vi "driveLoadingStationToCargoShipSM.vi"(9 "Initialized":bool) -> (2 "Drive State":T1)   [LabVIEW 2018]
uses:
  driveStateEnum.ctl
  driveLoadingStationToCargoShipEnum.ctl
  MotionProfile/Constants.vi
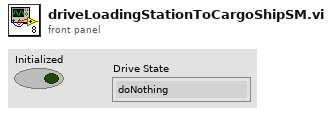
[diagram p1: front panel]
types:
  T1 = typedef "driveStateEnum.ctl" = enum16{"doNothing", "Manuel", "Teleop", "Follow Path (init)", "Follow Path", "Move to Target", "Climb", "Line Align", "Rotate180", "Align50Degrees"}
  T2 = typedef "driveLoadingStationToCargoShipEnum.ctl" = enum16{"1 - MP Back Up (init)", "2 - MP Back Up", "3 - Spin", "4 - MP Goto Cargo (init)", "5 - MP Goto Cargo", "6 - doNothing"}
  T3 = typedef "WPI_MotorControlDeviceRef.ctl" = cluster{"DeviceStatus":errorcluster, "Type":T4, "PWM":cluster{"PWM Channel":T5, "DeadBand":T6}, "CAN":cluster{"Device Number":u8, "SetOutput VI Ref":variant, "GetOutput VI Ref":variant, "Enable VI Ref":variant, "Disable VI Ref":variant, "Data":variant}, "Invert":bool, "DIO PWM":cluster{"PWM \"Enable\" Channel":T5, "DIOChannel":T7, "PWM Rate":dbl}}
  T4 = typedef "WPI_MotorControlType.ctl" = enum16{"PWM", "CAN", "DIO PWM"}
  T5 = typedef "FPGA_DIOPWMChannel.ctl" = enum8{"PWM 0", "PWM 1", "PWM 2", "PWM 3", "PWM 4", "PWM 5", "PWM 6", "PWM 7", "PWM 8", "PWM 9", "PWM MXP 0", "PWM MXP 1", "PWM MXP 2", "PWM MXP 3", "PWM MXP 4", "PWM MXP 5", "PWM MXP 6", "PWM MXP 7", "PWM MXP 8", "PWM MXP 9", "Invalid"}
  T6 = typedef "WPI_PWMDeadband.ctl" = cluster{"Name":string, "maxPositivePwm":i32, "minPositivePwm":i32, "centerPwm":i32, "maxNegativePwm":i32, "minNegativePwm":i32, "angularRange":u16}
  T7 = typedef "FPGA_DIOChannel.ctl" = enum8{"DIO 0", "DIO 1", "DIO 2", "DIO 3", "DIO 4", "DIO 5", "DIO 6", "DIO 7", "DIO 8", "DIO 9", "DIO MXP 0", "DIO MXP 1", "DIO MXP 2", "DIO MXP 3", "DIO MXP 4", "DIO MXP 5", "DIO MXP 6", "DIO MXP 7", "DIO MXP 8", "DIO MXP 9", "DIO MXP 10", "DIO MXP 11", "DIO MXP 12", "DIO MXP 13", "DIO MXP 14", "DIO MXP 15", "SPI Port CS1", "SPI Port CS2", "SPI Port CS3", "SPI Port MISO", "SPI Port MOSI", "Invalid"}
  T8 = enum16{"[0, 360]", "[-180, 180]", "[0, 2PI]", "[-PI, PI]"}
  T9 = typedef "CTRE_PigeonIMU_DeviceRef.ctl" = cluster{"DeviceStatus":errorcluster, "Device Number":u8, "Type":T10, "Device ID":u32, "Handle":u64, "UsageFrame":u32, "Library Path":path}
  T10 = typedef "CTRE_PigeonIMU_ConnectionType.ctl" = u32
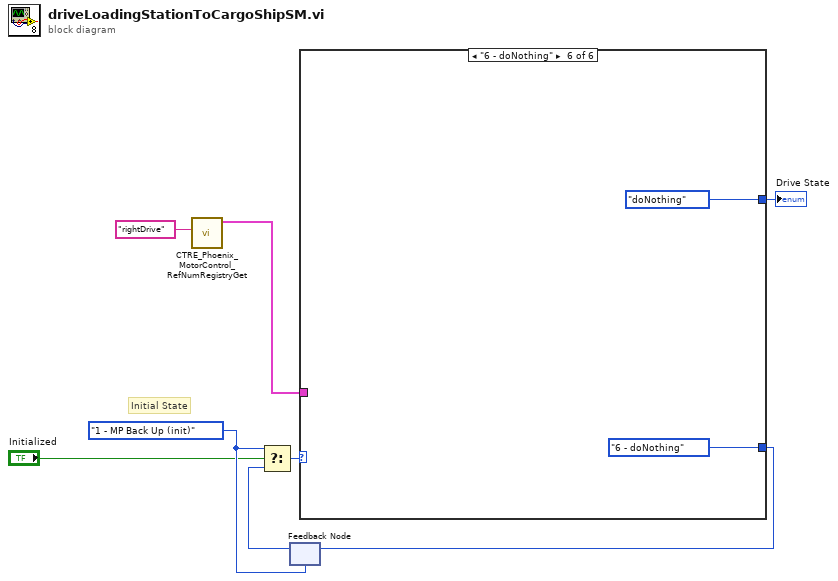
[diagram p0: block diagram]
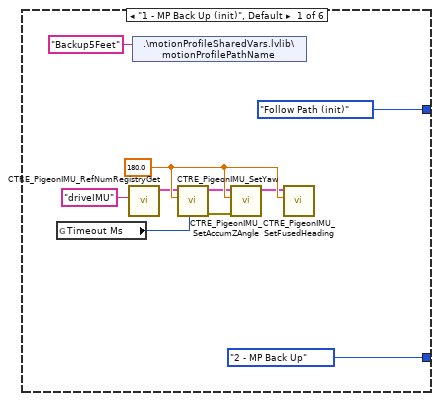
[diagram p2: hidden frame]
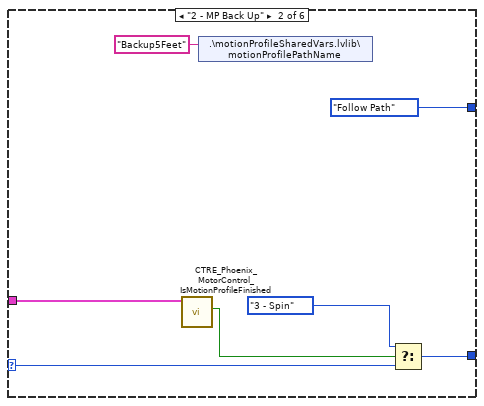
[diagram p3: hidden frame]
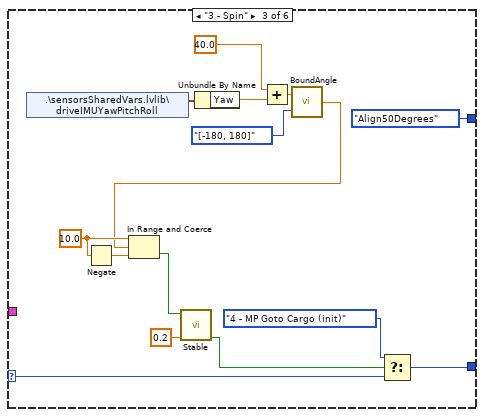
[diagram p4: hidden frame]
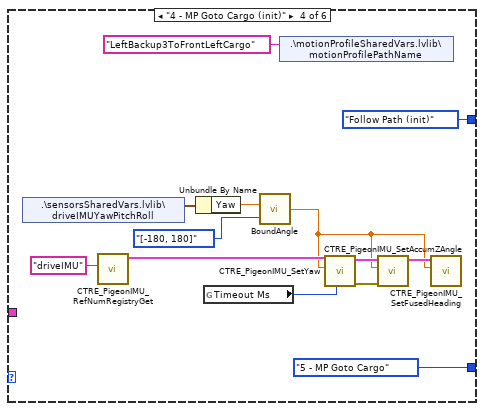
[diagram p5: hidden frame]
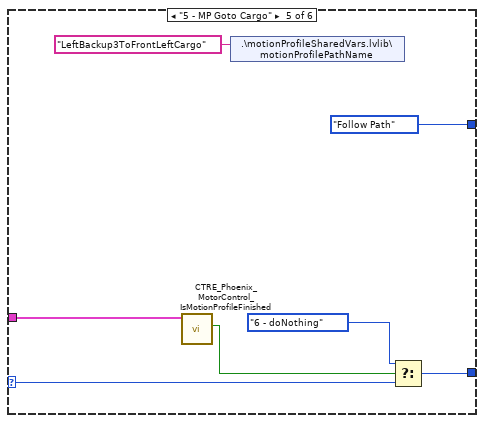
[diagram p6: hidden frame]
diagram:
  w6 = driveLoadingStationToCargoShipEnum."1 - MP Back Up (init)"
  # "Initial State"
  n1 = call <vilib>:"CTRE_Phoenix_MotorControl_RefNumRegistryGet.vi"("refnum name"="rightDrive") -> ("PhoenixMotorControlDevRef"=w3:T3)  [unwired: 9 in, 1 out]
  n2 = feedback #1(w6) -> (w7:T2)
  n3 = Select(t=w6, s="Initialized", f=w7) -> (s? t:f=w8:T2)
  n4 = case shown="\"6 - doNothing\"" w8 {
    selector: w8 -> [_ w20 w40 _ w55 _]
    tunnel: [driveLoadingStationToCargoShipEnum."2 - MP Back Up" w24 w39 driveLoadingStationToCargoShipEnum."5 - MP Goto Cargo" w59 driveLoadingStationToCargoShipEnum."6 - doNothing"] -> w5
    tunnel: [driveStateEnum."Follow Path (init)" ("Drive State Enum") driveStateEnum."Follow Path" ("Drive State Enum") driveStateEnum."Align50Degrees" ("Drive State Enum") driveStateEnum."Follow Path (init)" ("Drive State Enum") driveStateEnum."Follow Path" ("Drive State Enum") driveStateEnum."doNothing" ("Drive State Enum")] -> w1
    tunnel: w3 -> [_ w22 _ _ w57 _]
    frame "1 - MP Back Up (init)", Default {
      w15 = 180.0 ("Angle (Deg)")
      n5 = global read "Constants.vi" "Timeout Ms"() -> (w12:i32)
      n6 = call <vilib>:"CTRE_PigeonIMU_RefNumRegistryGet.vi"("refnum name"="driveIMU") -> ("PigeonIMUDevRef"=w9:T9)  [unwired: 9 in, 1 out]
      n7 = shared-variable ".\\motionProfileSharedVars.lvlib\\motionProfilePathName"("Backup5Feet" ("motionProfilePathName")) -> ()  [unwired: 1 in, 1 out]
      n8 = call <vilib>:"CTRE_PigeonIMU_SetYaw.vi"("timeoutMs"=w12, "Value"=w15, "PigeonIMUDevRef"=w9) -> ("error out"=w10:errorcluster, "PigeonIMUDevRef"=w11:T9)  [unwired: 7 in]
      n9 = call <vilib>:"CTRE_PigeonIMU_SetAccumZAngle.vi"("error in (no error)"=w10, "Angle (Deg)"=w15, "PigeonIMUDevRef"=w11) -> ("PigeonIMUDevRef"=w13:T9)  [unwired: 7 in, 1 out]
      n10 = call <vilib>:"CTRE_PigeonIMU_SetFusedHeading.vi"("Value"=w15, "PigeonIMUDevRef 2"=w13) -> ()  [unwired: 8 in, 2 out]
    }
    frame "2 - MP Back Up" {
      n11 = call <vilib>:"CTRE_Phoenix_MotorControl_IsMotionProfileFinished.vi"("PhoenixMotorControlDevRef"=w22) -> ("Is Motion Profile Finished?"=w21:bool)  [unwired: 8 in, 2 out]
      n12 = shared-variable ".\\motionProfileSharedVars.lvlib\\motionProfilePathName"("Backup5Feet" ("motionProfilePathName")) -> ()  [unwired: 1 in, 1 out]
      n13 = Select(t=driveLoadingStationToCargoShipEnum."3 - Spin", s=w21, f=w20) -> (s? t:f=w24:T2)
    }
    frame "3 - Spin" {
      w33 = 10.0 ("upper limit")
      n14 = shared-variable ".\\sensorsSharedVars.lvlib\\driveIMUYawPitchRoll"() -> (w32:cluster{"Yaw":dbl, "Pitch":dbl, "Roll":dbl})  [unwired: 1 in, 1 out]
      n15 = Negate(x=w33) -> (-x=w34:dbl)
      n16 = Unbundle By Name(w32) -> ("Yaw"=w27:dbl)
      n17 = Add(x=40.0 ("y"), y=w27) -> (x+y=w28:dbl)
      n18 = call <userlib>:"BoundAngle.vi"("Type"=T8."[-180, 180]", "Angle"=w28) -> ("Bound Angle"=w29:dbl)
      n19 = In Range and Coerce(upper limit=w33, x=w29, lower limit=w34) -> (In Range?=w35:bool)  [unwired: 1 out]
      n20 = call <userlib>:"Stable.vi"("Eval Period (sec)"=0.2, "Signal Input"=w35) -> ("Stable"=w37:bool)  [unwired: 9 in]
      n21 = Select(t=driveLoadingStationToCargoShipEnum."4 - MP Goto Cargo (init)", s=w37, f=w40) -> (s? t:f=w39:T2)
    }
    frame "4 - MP Goto Cargo (init)" {
      n22 = shared-variable ".\\sensorsSharedVars.lvlib\\driveIMUYawPitchRoll"() -> (w44:cluster{"Yaw":dbl, "Pitch":dbl, "Roll":dbl})  [unwired: 1 in, 1 out]
      n23 = call <vilib>:"CTRE_PigeonIMU_RefNumRegistryGet.vi"("refnum name"="driveIMU") -> ("PigeonIMUDevRef"=w45:T9)  [unwired: 9 in, 1 out]
      n24 = Unbundle By Name(w44) -> ("Yaw"=w42:dbl)
      n25 = global read "Constants.vi" "Timeout Ms"() -> (w48:i32)
      n26 = call <userlib>:"BoundAngle.vi"("Type"=T8."[-180, 180]", "Angle"=w42) -> ("Bound Angle"=w41:dbl)
      n27 = shared-variable ".\\motionProfileSharedVars.lvlib\\motionProfilePathName"("LeftBackup3ToFrontLeftCargo" ("motionProfilePathName")) -> ()  [unwired: 1 in, 1 out]
      n28 = call <vilib>:"CTRE_PigeonIMU_SetYaw.vi"("timeoutMs"=w48, "Value"=w41, "PigeonIMUDevRef"=w45) -> ("error out"=w46:errorcluster, "PigeonIMUDevRef"=w47:T9)  [unwired: 7 in]
      n29 = call <vilib>:"CTRE_PigeonIMU_SetAccumZAngle.vi"("error in (no error)"=w46, "Angle (Deg)"=w41, "PigeonIMUDevRef"=w47) -> ("PigeonIMUDevRef"=w49:T9)  [unwired: 7 in, 1 out]
      n30 = call <vilib>:"CTRE_PigeonIMU_SetFusedHeading.vi"("Value"=w41, "PigeonIMUDevRef 2"=w49) -> ()  [unwired: 8 in, 2 out]
    }
    frame "5 - MP Goto Cargo" {
      n31 = call <vilib>:"CTRE_Phoenix_MotorControl_IsMotionProfileFinished.vi"("PhoenixMotorControlDevRef"=w57) -> ("Is Motion Profile Finished?"=w56:bool)  [unwired: 8 in, 2 out]
      n32 = shared-variable ".\\motionProfileSharedVars.lvlib\\motionProfilePathName"("LeftBackup3ToFrontLeftCargo" ("motionProfilePathName")) -> ()  [unwired: 1 in, 1 out]
      n33 = Select(t=driveLoadingStationToCargoShipEnum."6 - doNothing", s=w56, f=w55) -> (s? t:f=w59:T2)
    }
    frame "6 - doNothing" {
    }
  }
  "Drive State" <- w1
  n34 = feedback-in #1(w5) -> ()
